vi "updatePayload.vi"(7 "path in":path=path "C:/dev/Hexagon-VTD-Custom-Device/Libraries/VC.dll", 8 "error in (no error)":errorcluster, 10 "payload":u8[](array[numeric]), 11 "paeseHandle in":u64) -> (0 "error out":errorcluster, 1 "simFrame":dbl, 2 "simTime":dbl, 3 "paeseHandle out":u64, 5 "isComplete":u8)   [LabVIEW 2023, in "RDB.lvlib"]
uses:
  RDB.lvlib
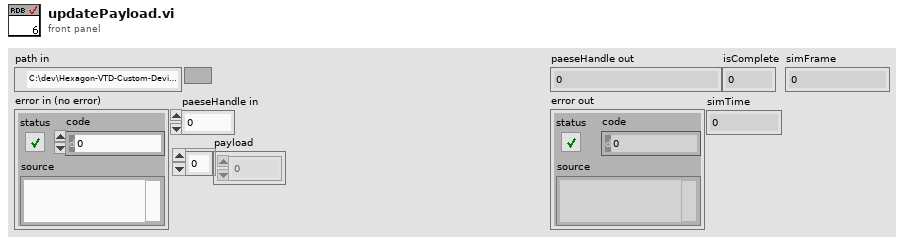
[diagram p1: front panel]
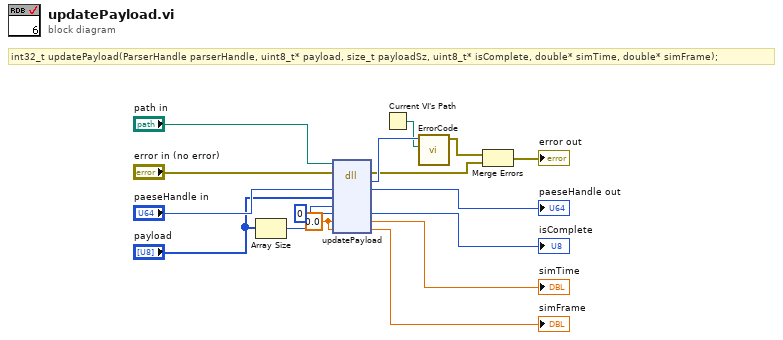
[diagram p0: block diagram]
diagram:
  w5 = 0.0 ("simTime")
  # "int32_t updatePayload(ParserHandle parserHandle, uint8_t* payload, size_t payloadSz, uint8_t* isComplete, double* simTime, double* simFrame);"
  n1 = Array Size(array="payload") -> (size(s)=w7:i32)
  n2 = dll-call lib="C:/dev/Hexagon-VTD-Custom-Device/Libraries/VC.dll" fn="updatePayload"(path in="path in", error in="error in (no error)", "paeseHandle"="paeseHandle in", "payload"="payload", "payloadSz"=w7, "isComplete"=u8 0, "simTime"=w5, "simFrame"=w5) -> (error out=w11:errorcluster, "return type"=w13:i32, "paeseHandle"=→"paeseHandle out":u64, "isComplete"=→"isComplete":u8, "simTime"=→"simTime":dbl, "simFrame"=→"simFrame":dbl)  [unwired: 3 in, 1 out]
  n3 = Current VI's Path() -> (path=w1:path)
  n4 = call "ErrorCode.vi"("parent VI path"=w1, "return type"=w13) -> ("error out"=w12:errorcluster)  [unwired: 9 in]
  n5 = Merge Errors(w12, w11) -> (→"error out":errorcluster)
